vi "LHPulse-11-15.vi"(2 "LHPulse(us)":T1, 3 "LHHeizen?":T2) -> ()   [LabVIEW 2010]
uses:
  <vilib>/eio/EIONode/EIONode.xnode
  <vilib>/rvi/eio/nirviEIOImplementation/nirviEIOImplementation.xnode
  <vilib>/rvi/eio/common/nirviEmuClasses.ctl
  <vilib>/rvi/eio/common/nirviEmuTemplateMethod_noerrors.vi
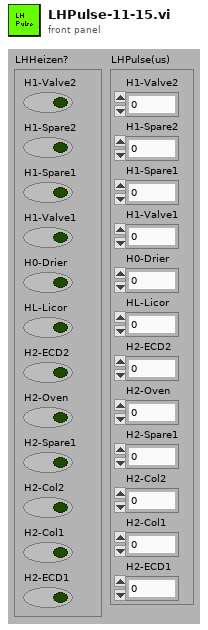
[diagram p1: front panel]
types:
  T1 = cluster{"H1-Valve2":u32, "H1-Spare2":u32, "H1-Spare1":u32, "H1-Valve1":u32, "H0-Drier":u32, "HL-Licor":u32, "H2-ECD2":u32, "H2-Oven":u32, "H2-Spare1":u32, "H2-Col2":u32, "H2-Col1":u32, "H2-ECD1":u32}
  T2 = cluster{"H1-Valve2":bool, "H1-Spare2":bool, "H1-Spare1":bool, "H1-Valve1":bool, "H0-Drier":bool, "HL-Licor":bool, "H2-ECD2":bool, "H2-Oven":bool, "H2-Spare1":bool, "H2-Col2":bool, "H2-Col1":bool, "H2-ECD1":bool}
  T3 = typedef "nirviEmuClasses.ctl" = enum16{"IO Read", "IO Write", "Method", "Property Read", "Property Write"}
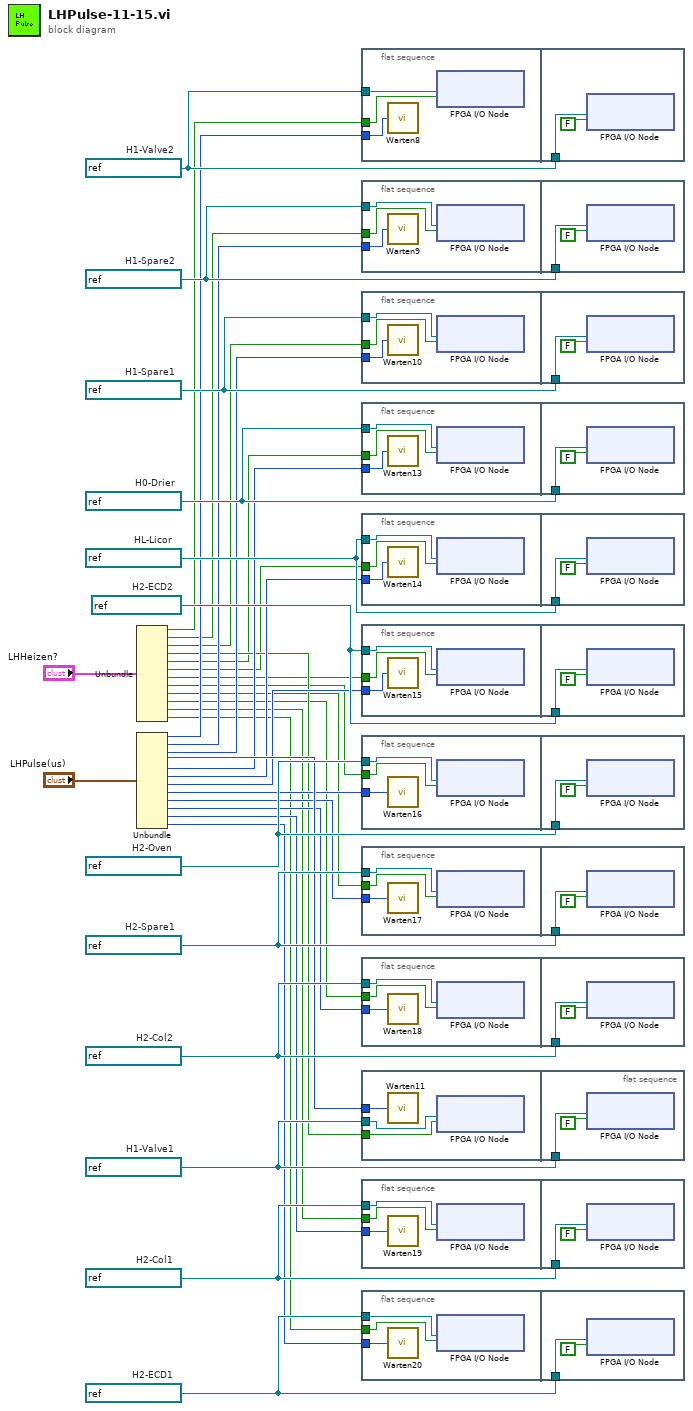
[diagram p0: block diagram]
diagram:
  w27 = refnum<k21> "Mod5/DIO20"  # H2-ECD1
  w28 = refnum<k21> "Mod5/DIO19"  # H2-Col1
  w29 = refnum<k21> "Mod5/DIO18"  # H2-Col2
  w30 = refnum<k21> "Mod5/DIO17"  # H2-Spare1
  w31 = refnum<k21> "Mod5/DIO16"  # H2-Oven
  w32 = refnum<k21> "Mod5/DIO1"  # H2-ECD2
  w33 = refnum<k21> "Mod5/DIO27"  # HL-Licor
  w34 = refnum<k21> "Mod5/DIO31"  # H0-Drier
  w35 = refnum<k21> "Mod6/DIO27"  # H1-Valve1
  w36 = refnum<k21> "Mod6/DIO26"  # H1-Spare1
  w37 = refnum<k21> "Mod6/DIO25"  # H1-Spare2
  w38 = refnum<k21> "Mod6/DIO24"  # H1-Valve2
  n1 = Unbundle("LHHeizen?") -> ("H1-Valve2"=w12:bool, "H1-Spare2"=w11:bool, "H1-Spare1"=w10:bool, "H1-Valve1"=w9:bool, "H0-Drier"=w8:bool, "HL-Licor"=w7:bool, "H2-ECD2"=w6:bool, "H2-Oven"=w5:bool, "H2-Spare1"=w4:bool, "H2-Col2"=w3:bool, "H2-Col1"=w2:bool, "H2-ECD1"=w1:bool)
  n2 = Unbundle("LHPulse(us)") -> ("H1-Valve2"=w24:u32, "H1-Spare2"=w23:u32, "H1-Spare1"=w22:u32, "H1-Valve1"=w21:u32, "H0-Drier"=w20:u32, "HL-Licor"=w19:u32, "H2-ECD2"=w18:u32, "H2-Oven"=w17:u32, "H2-Spare1"=w16:u32, "H2-Col2"=w15:u32, "H2-Col1"=w14:u32, "H2-ECD1"=w13:u32)
  n3 = flat-sequence {
    tunnel: w38 -> [w41]
    tunnel: w12 -> [w40]
    tunnel: w24 -> [w39]
    tunnel: w38 -> [w54]
    frame #0 {
      n4 = call "Warten8"("Count(uSec)"=w39) -> ()  [unwired: 1 out]
      n5 = xnode "FPGA I/O Node"("I/O Item"=w40, "FPGA I/O In"=w41) -> ()  [unwired: 1 out]
    }
    frame #1 {
      n6 = xnode "FPGA I/O Node"("I/O Item"=FALSE, "FPGA I/O In"=w54) -> ()  [unwired: 1 out]
    }
  }
  n7 = flat-sequence {
    tunnel: w37 -> [w68]
    tunnel: w11 -> [w67]
    tunnel: w23 -> [w66]
    tunnel: w37 -> [w81]
    frame #0 {
      n8 = call "Warten9"("Count(uSec)"=w66) -> ()  [unwired: 1 out]
      n9 = xnode "FPGA I/O Node"("I/O Item"=w67, "FPGA I/O In"=w68) -> ()  [unwired: 1 out]
    }
    frame #1 {
      n10 = xnode "FPGA I/O Node"("I/O Item"=FALSE, "FPGA I/O In"=w81) -> ()  [unwired: 1 out]
    }
  }
  n11 = flat-sequence {
    tunnel: w36 -> [w95]
    tunnel: w10 -> [w94]
    tunnel: w22 -> [w93]
    tunnel: w36 -> [w108]
    frame #0 {
      n12 = call "Warten10"("Count(uSec)"=w93) -> ()  [unwired: 1 out]
      n13 = xnode "FPGA I/O Node"("I/O Item"=w94, "FPGA I/O In"=w95) -> ()  [unwired: 1 out]
    }
    frame #1 {
      n14 = xnode "FPGA I/O Node"("I/O Item"=FALSE, "FPGA I/O In"=w108) -> ()  [unwired: 1 out]
    }
  }
  n15 = flat-sequence {
    tunnel: w34 -> [w122]
    tunnel: w8 -> [w121]
    tunnel: w20 -> [w120]
    tunnel: w34 -> [w135]
    frame #0 {
      n16 = call "Warten13"("Count(uSec)"=w120) -> ()  [unwired: 1 out]
      n17 = xnode "FPGA I/O Node"("I/O Item"=w121, "FPGA I/O In"=w122) -> ()  [unwired: 1 out]
    }
    frame #1 {
      n18 = xnode "FPGA I/O Node"("I/O Item"=FALSE, "FPGA I/O In"=w135) -> ()  [unwired: 1 out]
    }
  }
  n19 = flat-sequence {
    tunnel: w33 -> [w149]
    tunnel: w7 -> [w148]
    tunnel: w19 -> [w147]
    tunnel: w33 -> [w162]
    frame #0 {
      n20 = call "Warten14"("Count(uSec)"=w147) -> ()  [unwired: 1 out]
      n21 = xnode "FPGA I/O Node"("I/O Item"=w148, "FPGA I/O In"=w149) -> ()  [unwired: 1 out]
    }
    frame #1 {
      n22 = xnode "FPGA I/O Node"("I/O Item"=FALSE, "FPGA I/O In"=w162) -> ()  [unwired: 1 out]
    }
  }
  n23 = flat-sequence {
    tunnel: w32 -> [w176]
    tunnel: w6 -> [w175]
    tunnel: w18 -> [w174]
    tunnel: w32 -> [w189]
    frame #0 {
      n24 = call "Warten15"("Count(uSec)"=w174) -> ()  [unwired: 1 out]
      n25 = xnode "FPGA I/O Node"("I/O Item"=w175, "FPGA I/O In"=w176) -> ()  [unwired: 1 out]
    }
    frame #1 {
      n26 = xnode "FPGA I/O Node"("I/O Item"=FALSE, "FPGA I/O In"=w189) -> ()  [unwired: 1 out]
    }
  }
  n27 = flat-sequence {
    tunnel: w31 -> [w203]
    tunnel: w5 -> [w202]
    tunnel: w17 -> [w201]
    tunnel: w31 -> [w216]
    frame #0 {
      n28 = call "Warten16"("Count(uSec)"=w201) -> ()  [unwired: 1 out]
      n29 = xnode "FPGA I/O Node"("I/O Item"=w202, "FPGA I/O In"=w203) -> ()  [unwired: 1 out]
    }
    frame #1 {
      n30 = xnode "FPGA I/O Node"("I/O Item"=FALSE, "FPGA I/O In"=w216) -> ()  [unwired: 1 out]
    }
  }
  n31 = flat-sequence {
    tunnel: w30 -> [w230]
    tunnel: w4 -> [w229]
    tunnel: w16 -> [w228]
    tunnel: w30 -> [w243]
    frame #0 {
      n32 = call "Warten17"("Count(uSec)"=w228) -> ()  [unwired: 1 out]
      n33 = xnode "FPGA I/O Node"("I/O Item"=w229, "FPGA I/O In"=w230) -> ()  [unwired: 1 out]
    }
    frame #1 {
      n34 = xnode "FPGA I/O Node"("I/O Item"=FALSE, "FPGA I/O In"=w243) -> ()  [unwired: 1 out]
    }
  }
  n35 = flat-sequence {
    tunnel: w29 -> [w257]
    tunnel: w3 -> [w256]
    tunnel: w15 -> [w255]
    tunnel: w29 -> [w270]
    frame #0 {
      n36 = call "Warten18"("Count(uSec)"=w255) -> ()  [unwired: 1 out]
      n37 = xnode "FPGA I/O Node"("I/O Item"=w256, "FPGA I/O In"=w257) -> ()  [unwired: 1 out]
    }
    frame #1 {
      n38 = xnode "FPGA I/O Node"("I/O Item"=FALSE, "FPGA I/O In"=w270) -> ()  [unwired: 1 out]
    }
  }
  n39 = flat-sequence {
    tunnel: w35 -> [w284]
    tunnel: w9 -> [w283]
    tunnel: w21 -> [w282]
    tunnel: w35 -> [w297]
    frame #0 {
      n40 = call "Warten11"("Count(uSec)"=w282) -> ()  [unwired: 1 out]
      n41 = xnode "FPGA I/O Node"("I/O Item"=w283, "FPGA I/O In"=w284) -> ()  [unwired: 1 out]
    }
    frame #1 {
      n42 = xnode "FPGA I/O Node"("I/O Item"=FALSE, "FPGA I/O In"=w297) -> ()  [unwired: 1 out]
    }
  }
  n43 = flat-sequence {
    tunnel: w28 -> [w311]
    tunnel: w2 -> [w310]
    tunnel: w14 -> [w309]
    tunnel: w28 -> [w324]
    frame #0 {
      n44 = call "Warten19"("Count(uSec)"=w309) -> ()  [unwired: 1 out]
      n45 = xnode "FPGA I/O Node"("I/O Item"=w310, "FPGA I/O In"=w311) -> ()  [unwired: 1 out]
    }
    frame #1 {
      n46 = xnode "FPGA I/O Node"("I/O Item"=FALSE, "FPGA I/O In"=w324) -> ()  [unwired: 1 out]
    }
  }
  n47 = flat-sequence {
    tunnel: w27 -> [w338]
    tunnel: w1 -> [w337]
    tunnel: w13 -> [w336]
    tunnel: w27 -> [w351]
    frame #0 {
      n48 = call "Warten20"("Count(uSec)"=w336) -> ()  [unwired: 1 out]
      n49 = xnode "FPGA I/O Node"("I/O Item"=w337, "FPGA I/O In"=w338) -> ()  [unwired: 1 out]
    }
    frame #1 {
      n50 = xnode "FPGA I/O Node"("I/O Item"=FALSE, "FPGA I/O In"=w351) -> ()  [unwired: 1 out]
    }
  }
